vi "new_pigeon_status_period.vi"(8 "error in (no error)":errorcluster, 11 "PigeonIMUDevRef In":T1={"DeviceStatus"={"status"=FALSE, "code"=0, "source"=""}, "Device Number"=0, "Type"=352321536, "Device ID"=0, "Handle"=0, "UsageFrame"=0, "Library Path"=path ""} {"Type" items=["CAN"=352321536, "TalonSRX"=33554432]}) -> (0 "error out":errorcluster, 3 "PigeonIMUDevRef Out":T1={"DeviceStatus"={"status"=FALSE, "code"=0, "source"=""}, "Device Number"=0, "Type"=352321536, "Device ID"=0, "Handle"=0, "UsageFrame"=0, "Library Path"=path ""} {"Type" items=["CAN"=352321536, "TalonSRX"=33554432]})   [LabVIEW 2020]
uses:
  <vilib>/Rock Robotics/WPI/ThirdParty/Phoenix-LabVIEW/Pigeon IMU/CTRE_PigeonIMU_DeviceRef.ctl
  <vilib>/Rock Robotics/WPI/ThirdParty/Phoenix-LabVIEW/Pigeon IMU/CTRE_PigeonIMU_ConnectionType.ctl
  <vilib>/Rock Robotics/WPI/ThirdParty/Phoenix-LabVIEW/Pigeon IMU/CTRE_PigeonIMU_StatusFrameRate.ctl
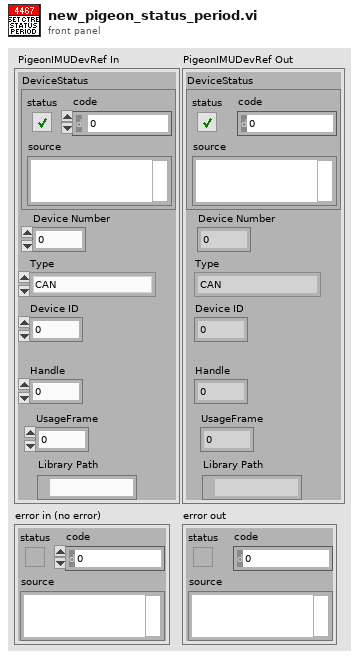
[diagram p1: front panel]
types:
  T1 = typedef "CTRE_PigeonIMU_DeviceRef.ctl" = cluster{"DeviceStatus":errorcluster, "Device Number":u8, "Type":T2, "Device ID":u32, "Handle":u64, "UsageFrame":u32, "Library Path":path}
  T2 = typedef "CTRE_PigeonIMU_ConnectionType.ctl" = u32
  T3 = typedef "CTRE_PigeonIMU_StatusFrameRate.ctl" = u32
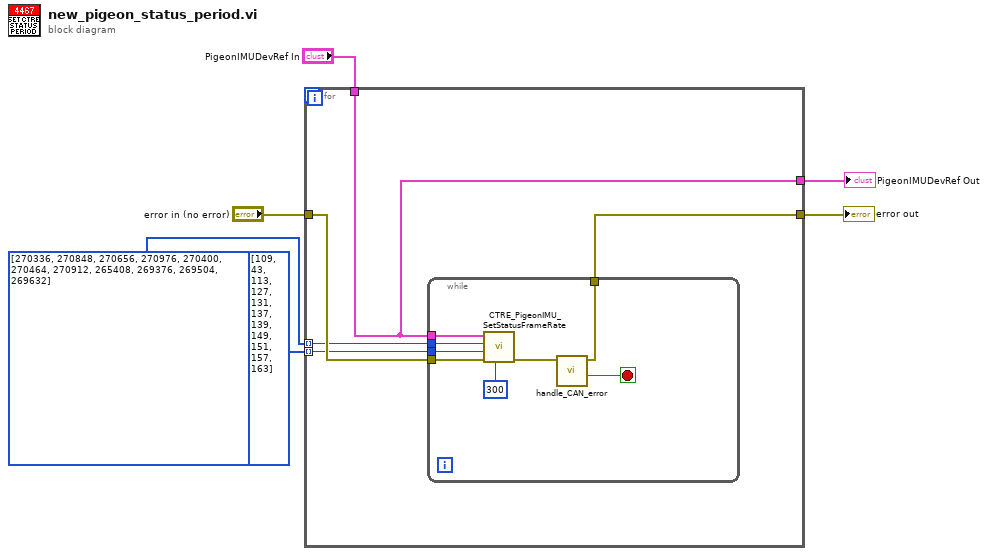
[diagram p0: block diagram]
diagram:
  w3 = T3[] [270336, 270848, 270656, 270976, 270400, 270464, 270912, 265408, 269376, 269504, 269632] items=["CondStatus_1_General"=270336, "CondStatus_9_SixDeg_YPR"=270848, "CondStatus_6_SensorFusion"=270656, "CondStatus_11_GyroAccum"=270976, "CondStatus_2_GeneralCompass"=270400, "CondStatus_3_GeneralAccel"=270464, "CondStatus_10_SixDeg_Quat"=270912, "RawStatus_4_Mag"=265408, "BiasedStatus_2_Gyro"=269376, "BiasedStatus_4_Mag"=269504, "BiasedStatus_6_Accel"=269632] ("StatusFrame")
  n1 = for {
    tunnel: [w11] -> w6
    tunnel: "PigeonIMUDevRef In" -> [w11]
    tunnel: w3 -> [w8] mode=indexing
    tunnel: i16[] [109, 43, 113, 127, 131, 137, 139, 149, 151, 157, 163] -> [w9] mode=indexing
    tunnel: "error in (no error)" -> [w10]
    tunnel: [w7] -> w5
    n2 = while {
      tunnel: w11 -> [w19]
      tunnel: w10 -> [w18]
      tunnel: w9 -> [w17]
      tunnel: w8 -> [w16]
      tunnel: [w12] -> w7
      stop <- w13 stop-if-true
      n3 = call <vilib>:"CTRE_PigeonIMU_SetStatusFrameRate.vi"("timeoutMs"=u32 300, "error in (no error)"=w18, "Period (ms)"=w17, "StatusFrame"=w16, "PigeonIMUDevRef"=w19) -> ("error out"=w14:errorcluster)  [unwired: 5 in, 1 out]
      n4 = call "handle_CAN_error.vi"("error in (no error)"=w14) -> ("stop"=w13:bool, "error out"=w12:errorcluster)  [unwired: 9 in]
    }
  }
  "error out" <- w5
  "PigeonIMUDevRef Out" <- w6
